vi "ForceAndPressureAhmed2.vi"() -> ()   [LabVIEW 2017]
uses:
  <vilib>/Analysis/NI_AALBase.lvlib
panel:
  out "Force Mean Convergence":dbl(graph)=0.23332198796908798
  out "Pressure Mean Convergence":dbl(graph)=0.00022051026462577283
  in  "Balance Check":i32
  in  "Tapping Check":i32=1
  in  "Time (s)":dbl=10.0 format="%#_13g"
  in  "Frequency (Hz)":dbl=1000.0 format="%#_13g"
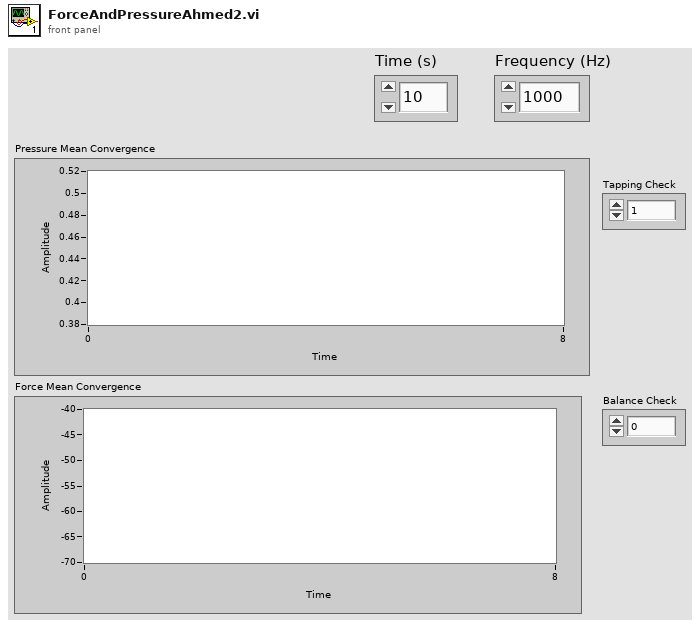
[diagram p1: front panel]
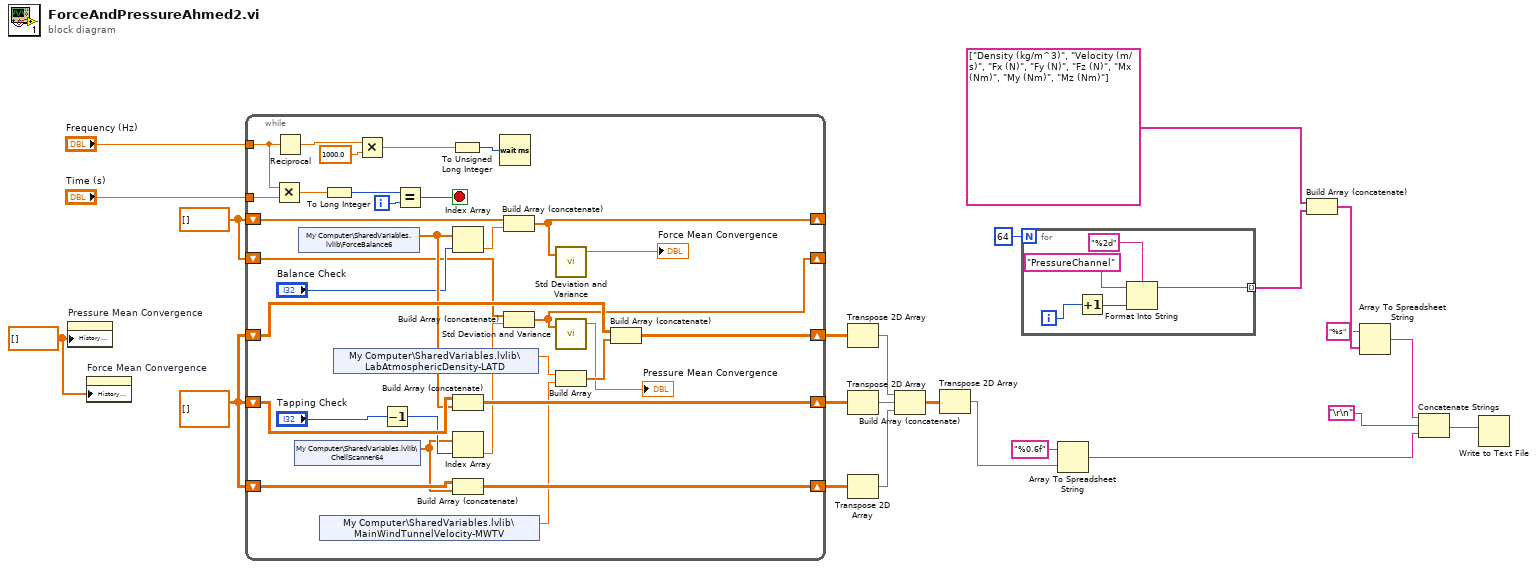
[diagram p0: block diagram]
diagram:
  w13 = dbl[] [] ("History Data")
  w20 = dbl[] []
  w21 = dbl[][] []
  n1 = property on="Pressure Mean Convergence" class="WFChart (strict)"("History Data"=w13) -> ()  [unwired: 2 in, 2 out]
  n2 = property on="Force Mean Convergence" class="WFChart (strict)"("History Data"=w13) -> ()  [unwired: 2 in, 2 out]
  n3 = while {
    tunnel: "Frequency (Hz)" -> [w51]
    tunnel: "Time (s)" -> [w50]
    shift-right: [w45] -> w17
    shift-left: w21 -> [w44]
    shift-right: [w46] -> w15
    shift-left: w21 -> [w43]
    shift-right: [w40] -> w19
    shift-left: w21 -> [w39]
    shift-right: [w32] -> _
    shift-left: w20 -> [w34]
    shift-right: [w28] -> _
    shift-left: w20 -> [w30]
    i -> [w33]
    stop <- w47 stop-if-true
    n4 = Multiply(x=w51, y=w50) -> (x*y=w49:dbl)
    n5 = Reciprocal(x=w51) -> (1/x=w55:dbl)
    n6 = shared-variable "My Computer\\SharedVariables.lvlib\\ChellScanner64"() -> (w25:dbl[])  [unwired: 1 in, 1 out]
    n7 = shared-variable "My Computer\\SharedVariables.lvlib\\ForceBalance6"() -> (w36:dbl[])  [unwired: 1 in, 1 out]
    n8 = shared-variable "My Computer\\SharedVariables.lvlib\\MainWindTunnelVelocity-MWTV"() -> (w24:dbl)  [unwired: 1 in, 1 out]
    n9 = To Long Integer(number=w49) -> (32bit integer=w48:i32)
    n10 = shared-variable "My Computer\\SharedVariables.lvlib\\LabAtmosphericDensity-LATD"() -> (w42:dbl)  [unwired: 1 in, 1 out]
    n11 = Multiply(x=w55, y=1000.0) -> (x*y=w54:dbl)
    n12 = Decrement(x="Tapping Check") -> (x-1=w37:i32)
    n13 = Equal?(x=w48, y=w33) -> (x = y?=w47:bool)
    n14 = To Unsigned Long Integer(number=w54) -> (unsigned 32bit integer=w53:u32)
    n15 = Index Array(array=w36, index="Balance Check") -> (element=w29:dbl)
    n16 = Build Array (concatenate)(w44, w36) -> (w45:dbl[][])
    n17 = Index Array(array=w25, index=w37) -> (element=w26:dbl)
    n18 = Build Array (concatenate)(w43, w25) -> (w46:dbl[][])
    n19 = Wait (ms)(milliseconds to wait=w53) -> ()  [unwired: 1 out]
    n20 = Build Array (concatenate)(w30, w29) -> (w28:dbl[])
    n21 = Build Array (concatenate)(w34, w26) -> (w32:dbl[])
    n22 = call <vilib>:"Std Deviation and Variance.vi"("X"=w28) -> ("mean"=→"Force Mean Convergence":dbl)  [unwired: 1 in, 2 out]
    n23 = call <vilib>:"Std Deviation and Variance.vi"("X"=w32) -> ("mean"=→"Pressure Mean Convergence":dbl)  [unwired: 1 in, 2 out]
    n24 = Build Array(w42, w24) -> (w41:dbl[])
    n25 = Build Array (concatenate)(w39, w41) -> (w40:dbl[][])
  }
  n26 = Transpose 2D Array(2D array=w19) -> (transposed array=w18:dbl[][])
  n27 = Transpose 2D Array(2D array=w17) -> (transposed array=w16:dbl[][])
  n28 = Transpose 2D Array(2D array=w15) -> (transposed array=w14:dbl[][])
  n29 = Build Array (concatenate)(w18, w16, w14) -> (w2:dbl[][])
  n30 = Transpose 2D Array(2D array=w2) -> (transposed array=w1:dbl[][])
  n31 = for {
    N: 64 -> [_]
    tunnel: [w56] -> w10 mode=indexing
    i -> [w60]
    n32 = Increment(x=w60) -> (x+1=w59:i32)
    n33 = Format Into String(format string="%2d", initial string="PressureChannel", w59) -> (resulting string=w56:string)  [unwired: 1 in, 1 out]
  }
  n34 = Array To Spreadsheet String(array=w1, 3:"%0.6f" ("format string")) -> (spreadsheet string=w7:string)  [unwired: 1 in]
  n35 = Build Array (concatenate)(string[] ["Density (kg/m^3)", "Velocity (m/s)", "Fx (N)", "Fy (N)", "Fz (N)", "Mx (Nm)", "My (Nm)", "Mz (Nm)"], w10) -> (w9:string[])
  n36 = Array To Spreadsheet String(array=w9, 3:"%s" ("format string")) -> (spreadsheet string=w8:string)  [unwired: 1 in]
  n37 = Concatenate Strings(w8, "\r\n", w7) -> (w5:string)
  n38 = Write to Text File(text=w5) -> ()  [unwired: 3 in, 3 out]
